vi "Digitizer Clock In Data Secondary.vi"(6 "Digitize Read Delay Ticks":u32, 9 "Digitize # Bits":u32=16, 10 "Convert Clock Ticks":u32=20, 11 "Refnum in":refnum<k21>) -> (3 "Data Out":T1)   [LabVIEW 2017]
doc: "Author: Scott Hannahs <sth@magnet.fsu.edu>\nCopyright 2018 Florida State University, All rights reserved."
uses:
  <vilib>/eio/EIONode/EIONode.xnode
  <vilib>/rvi/eio/common/nirviEmuTemplateMethod_errors.vi
  SCH Data Controls/SCH Raw Int Data Secondary.ctl
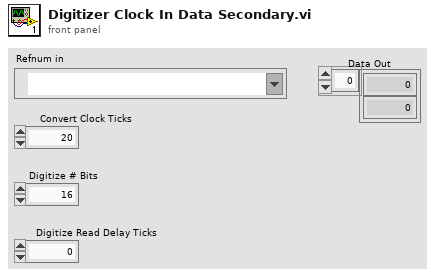
[diagram p1: front panel]
types:
  T1 = typedef "SCH Raw Int Data Secondary.ctl" = i16[]
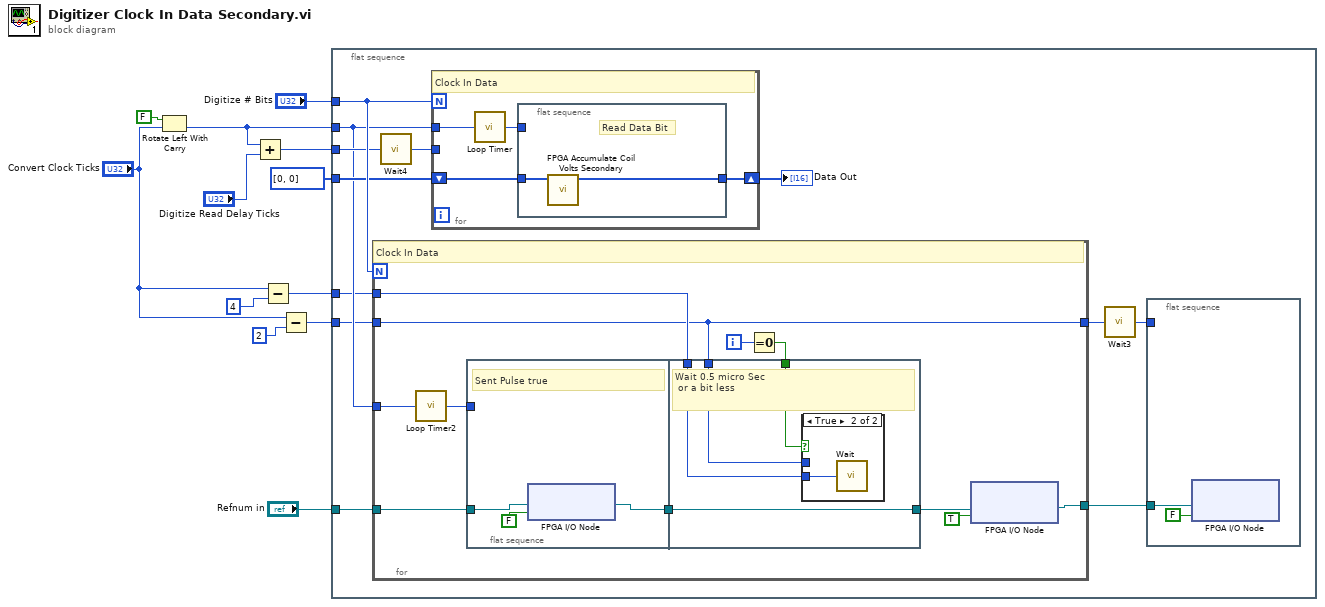
[diagram p0: block diagram]
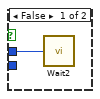
[diagram p2: hidden frame]
diagram:
  n1 = Rotate Left With Carry(2:"Convert Clock Ticks", 3:FALSE ("carry")) -> (0:w3:u32)  [unwired: 1 out]
  n2 = Add(x=w3, y="Digitize Read Delay Ticks") -> (x+y=w7:u32)
  n3 = Subtract(x="Convert Clock Ticks", y=u32 4) -> (x-y=w1:u32)
  n4 = Subtract(x="Convert Clock Ticks", y=u32 2) -> (x-y=w2:u32)
  n5 = flat-sequence {
    tunnel: "Digitize # Bits" -> [w24]
    tunnel: w7 -> [w22]
    tunnel: T1 [0, 0] ("Data Array In") -> [w21]
    tunnel: "Refnum in" -> [w20]
    tunnel: w3 -> [w19]
    tunnel: w2 -> [w15]
    tunnel: w1 -> [w18]
    frame #0 {
      n6 = for {
        N: w24 -> [_]
        tunnel: w20 -> [w39]
        tunnel: w19 -> [w38]
        tunnel: w15 -> [w33]
        tunnel: w18 -> [w35]
        tunnel: [w34] -> w17
        tunnel: [w33] -> w14
        i -> [w37]
        # "Clock In Data"
        n7 = call "Loop Timer2"("Count(Ticks)"=w38) -> ("Tick Count(Ticks)"=w42:u32)
        n8 = flat-sequence {
          tunnel: w42 -> [_]
          tunnel: w39 -> [w45]
          tunnel: [w44] -> w43
          tunnel: [w50] -> w41
          tunnel: w43 -> [w50]
          tunnel: w36 -> [w49]
          tunnel: w33 -> [w48]
          tunnel: w35 -> [w47]
          frame #0 {
            # "Sent Pulse true"
            n9 = xnode "FPGA I/O Node"("I/O Item"=FALSE ("Connector0/DIO0"), "FPGA I/O In"=w45) -> ("FPGA I/O Out"=w44:refnum<k21>)
          }
          frame #1 {
            # "Wait 0.5 micro Sec\n or a bit less"
            n10 = case shown="True" w49 {
              tunnel: w48 -> [w51 _]
              tunnel: w47 -> [_ w52]
              frame False {
                n11 = call "Wait2"("Count(Ticks)"=w51) -> ()  [unwired: 1 out]
              }
              frame True {
                n12 = call "Wait"("Count(Ticks)"=w52) -> ()  [unwired: 1 out]
              }
            }
          }
        }
        n13 = Equal To 0?(x=w37) -> (x = 0?=w36:bool)
        n14 = xnode "FPGA I/O Node"("I/O Item"=TRUE ("Connector0/DIO0"), "FPGA I/O In"=w41) -> ("FPGA I/O Out"=w34:refnum<k21>)  [unwired: 1 in, 1 out]
      }
      n15 = call "Wait4"("Count(Ticks)"=w22) -> ("Tick Count(Ticks)"=w23:u32)
      n16 = for {
        N: w24 -> [_]
        shift-right: [w30] -> w13
        shift-left: w21 -> [w29]
        tunnel: w23 -> [_]
        tunnel: w19 -> [w27]
        # "Clock In Data"
        n17 = call "Loop Timer"("Count(Ticks)"=w27) -> ("Tick Count(Ticks)"=w28:u32)
        n18 = flat-sequence {
          tunnel: [w32] -> w30
          tunnel: w29 -> [w31]
          tunnel: w28 -> [_]
          frame #0 {
            # "Read Data Bit"
            n19 = call "FPGA Accumulate Coil Volts Secondary.vi"("Data Array In"=w31) -> ("Data Array Out"=w32:T1)  [unwired: 10 in]
          }
        }
      }
      "Data Out" <- w13
      n20 = call "Wait3"("Count(Ticks)"=w14) -> ("Tick Count(Ticks)"=w16:u32)
      n21 = flat-sequence {
        tunnel: w17 -> [w26]
        tunnel: w16 -> [_]
        frame #0 {
          n22 = xnode "FPGA I/O Node"("I/O Item"=FALSE, "FPGA I/O In"=w26) -> ()  [unwired: 1 in, 2 out]
        }
      }
    }
  }
